vi "error_processor.vi"(8 "error in (no error)":errorcluster) -> (0 "error out":errorcluster)   [LabVIEW 2021]
uses:
  FGVs/FGVstates.ctl
  <vilib>/Utility/error.llb/DialogType.ctl
  FGVs/AppStates.ctl
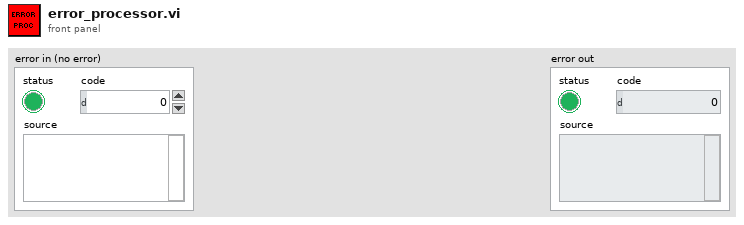
[diagram p1: front panel]
types:
  T1 = typedef "FGVstates.ctl" = enum16{"Init", "Set", "Get", "De-Init"}
  T2 = typedef "data_exchange_fgv.ctl" = cluster{"queue states":refnum<queue>, "audio data":refnum<queue>, "error queue":refnum<queue>}
  T3 = typedef "AppStates.ctl" = enum16{"Init", "Scan Music Dir", "Idle", "Playback", "Enqueue samples", "Pause playback", "Stop playback", "Exit"}
  T4 = typedef "DialogType.ctl" = u16
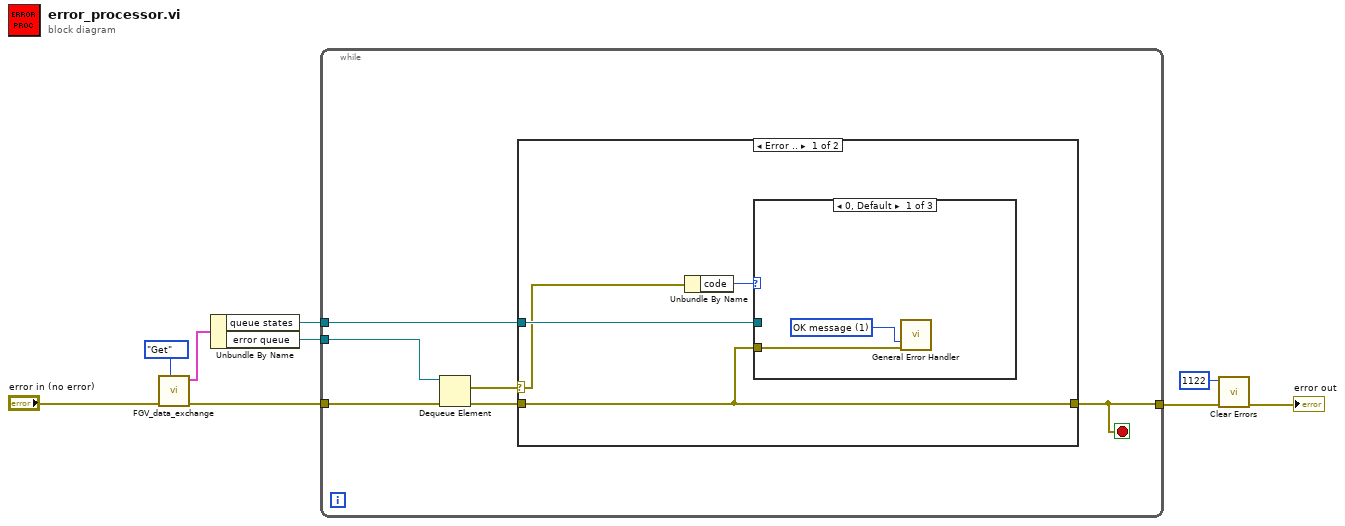
[diagram p0: block diagram]
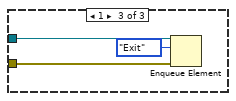
[diagram p3: hidden frame]
diagram:
  n1 = call "FGV_data_exchange.vi"("FGV states"=FGVstates."Get", "error in (no error)"="error in (no error)") -> ("error out"=w8:errorcluster, "main_cycle_queue"=w7:T2)  [unwired: 8 in]
  n2 = Unbundle By Name(w7) -> ("queue states"=w5:refnum<queue>, "error queue"=w6:refnum<queue>)
  n3 = while {
    tunnel: w8 -> [w15]
    tunnel: w6 -> [w12]
    tunnel: w5 -> [w11]
    tunnel: [w10] -> w4
    stop <- w10 stop-if-true
    n4 = Dequeue Element(queue=w12, error in (no error)=w15) -> (element=w13:errorcluster, error out=w14:errorcluster)  [unwired: 1 in, 2 out]
    n5 = case shown="Error .." w13 {
      selector: w13 -> [w16 _]
      tunnel: w14 -> [w18 w25]
      tunnel: [w18 w25] -> w10
      tunnel: w11 -> [w19 _]
      frame Error {
        n6 = Unbundle By Name(w16) -> ("code"=w17:i32)
        n7 = case shown="0, Default" w17 {
          tunnel: w19 -> [_ _ w24]
          tunnel: w18 -> [w21 _ w23]
          frame 0, Default {
            w20 = T4 1 items=["no dialog", "OK message", "continue or stop message", "OK message + warnings", "continue/stop + warnings"] ("type of dialog (OK msg:1)")
            n8 = call <vilib>:"General Error Handler.vi"("type of dialog (OK msg:1)"=w20, "error in (no error)"=w21) -> ()  [unwired: 9 in, 5 out]
          }
          frame 4805 {
          }
          frame 1 {
            n9 = Enqueue Element(queue=w24, element=AppStates."Exit", error in (no error)=w23) -> ()  [unwired: 1 in, 3 out]
          }
        }
      }
      frame No Error {
      }
    }
  }
  n10 = call <vilib>:"Clear Errors.vi"("error in (no error)"=w4, "specific error code to clear (0: all)"=1122) -> ("error out"=→"error out":errorcluster)  [unwired: 4 in, 1 out]
